vi "[GV]_GPS Validity.vi"() -> ()   [LabVIEW 2016]
panel:
  out "GPS Validity":bool
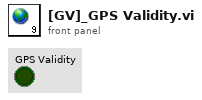
[diagram p1: front panel]
diagram:
